vi "Band Magnitude - Peak (Frequency).vi"(0 "power spectrum [EU^2 rms]":cluster{"f0":dbl, "df":dbl, "magnitude":sgl[]} {"magnitude" format="%.2p"; "df" format="%.2p"; "f0" format="%.2p"}, 5 "Start":dbl, 7 "Stop":dbl=1000.0 format="%#_13g", 11 "error in (no error)":errorcluster) -> (6 "Max Peak in Band [EU rms]":sgl, 15 "error out":errorcluster)   [LabVIEW 2017, in "VibrationAnalysisFunctions.lvlib"]
uses:
  <vilib>/addons/InsightCM/Utilities/Analysis/Vibration/VibrationAnalysisFunctions.lvlib
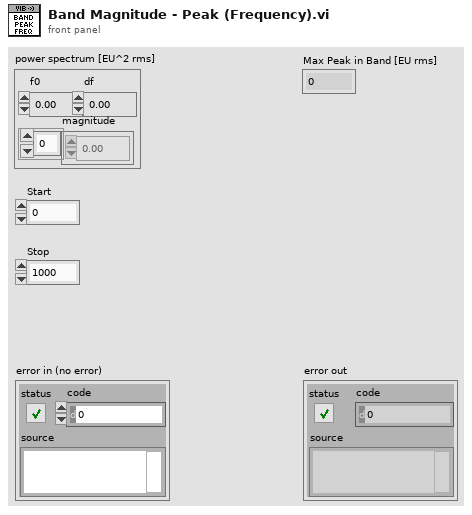
[diagram p1: front panel]
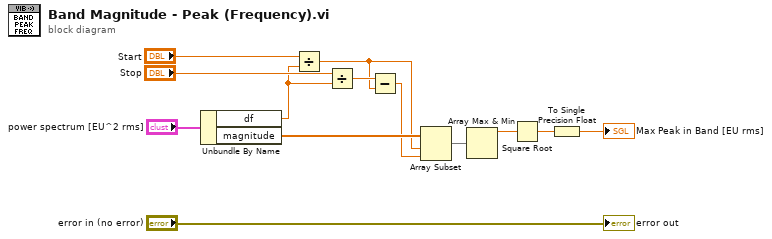
[diagram p0: block diagram]
diagram:
  n1 = Unbundle By Name("power spectrum [EU^2 rms]") -> ("df"=w8:dbl, "magnitude"=w11:sgl[])
  n2 = Divide(x="Start", y=w8) -> (x/y=w5:dbl)
  n3 = Divide(x="Stop", y=w8) -> (x/y=w7:dbl)
  n4 = Subtract(x=w7, y=w5) -> (x-y=w6:dbl)
  n5 = Array Subset(array=w11, index=w5, length=w6) -> (w4:sgl[])
  n6 = Array Max & Min(array=w4) -> (max value=w3:sgl)  [unwired: 3 out]
  n7 = Square Root(x=w3) -> (sqrt(x)=w1:sgl)
  n8 = To Single Precision Float(number=w1) -> (single precision float=→"Max Peak in Band [EU rms]":sgl)
  "error out" <- "error in (no error)"
